vi "Launcher.vi"() -> ()   [LabVIEW 2023]
uses:
  Workers/Table/Table.lvclass
  <vilib>/addons/_Workers/Debugger/Debug Client/Debug Client.lvlib
  C:/Program Files (x86)/National Instruments/LabVIEW 2023/vi.lib/addons/_Workers/Library/Classes/Worker/Worker.lvclass
panel:
  in  "# Philosophers":i32=5 min=5 max=500 step=1
  # "Overview:  https://en.wikipedia.org/wiki/Dining_philosophers_problem\n\nRequirements:  LabVIEW 2023 Q1   Workers SDK by Scarfe Controls\n\n                              https://www.workersforlabview.com/\n\nInstructions:  Run the VI."
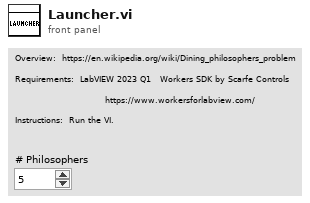
[diagram p1: front panel]
types:
  T1 = enum32{"Invalid", "Standard", "Closed", "Hidden", "Minimized", "Maximized"}
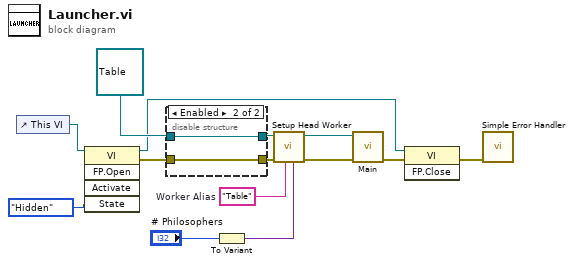
[diagram p0: block diagram]
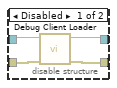
[diagram p2: hidden frame]
diagram:
  w12 = "Table"  # Worker Alias
  n1 = control-ref of="This VI"() -> (w7:refnum<vi>)
  n2 = invoke class="VI" method="FP.Open"(reference=w7, "State"=T1."Hidden") -> (reference out=w4:refnum<vi>, error out=w8:errorcluster)  [unwired: 3 in, 3 out]
  n3 = disable-structure shown="Enabled" {
    disable-tunnel: [w18 w20] -> w11
    disable-tunnel: refnum<class "Table.lvclass"> refnum ("Worker User Object") -> [w17 w19]
    disable-tunnel: [w16 w19] -> w9
    disable-tunnel: w8 -> [w15 w20]
    frame Disabled {
      n4 = call <vilib>:"Debug Client Loader.vi"("error in (no error)"=w15, "Worker"=w17) -> ("error out"=w18:errorcluster, "Worker out"=w16:refnum<class "Table.lvclass">)  [unwired: 8 in]
    }
    frame Enabled {
    }
  }
  n5 = To Variant(anything="# Philosophers") -> (Variant=w1:variant)
  n6 = call-dynamic "Setup Head Worker.vi"("Initalization Data"=w1, "Worker Alias"=w12, "error in"=w11, "Worker"=w9) -> ("error out"=w14:errorcluster, "Worker out"=w13:refnum<class "Table.lvclass">)  [unwired: 6 in]
  n7 = call-dynamic "Main.vi"("error in"=w14, "Table in"=w13) -> ("error out"=w6:errorcluster)  [unwired: 8 in, 1 out]
  n8 = invoke class="VI" method="FP.Close"(reference=w4, error in=w6) -> (error out=w5:errorcluster)  [unwired: 1 in, 2 out]
  n9 = call <vilib>:"Simple Error Handler.vi"("error in (no error)"=w5) -> ()  [unwired: 4 in, 5 out]
